vi "AddToCollection.vi"(8 "error in (no error)":errorcluster, 10 "IRenderable":refnum<class "IRenderable.lvclass">, 11 "Collection in":refnum<class "Collection.lvclass">) -> (0 "error out":errorcluster, 3 "Collection out":refnum<class "Collection.lvclass">)   [LabVIEW 2021, in "Markdown.lvlib" / "Collection.lvclass"]
uses:
  Collection.lvclass
  IRenderable/IRenderable.lvclass
  Collection.lvclass/Collection.ctl
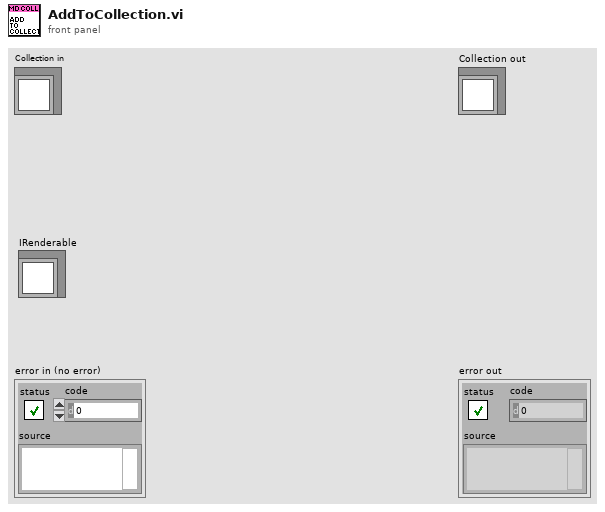
[diagram p1: front panel]
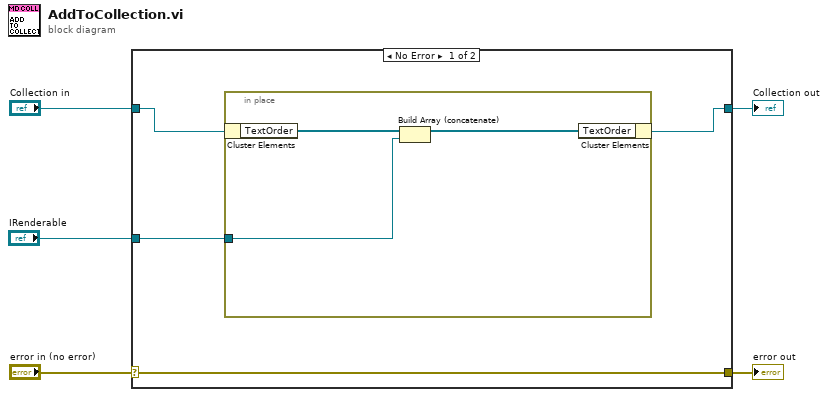
[diagram p0: block diagram]
diagram:
  n1 = case shown="No Error" "error in (no error)" {
    selector: "error in (no error)" -> [w9 w14]
    tunnel: [w9 w14] -> w4
    tunnel: [w6 w13] -> w2
    tunnel: "Collection in" -> [w8 w13]
    tunnel: "IRenderable" -> [w7 _]
    frame No Error {
      n2 = in-place {
        in-place-border: w7 -> [w10]
        n3 = in-place-cluster #1(w8) -> ("TextOrder"=w12:refnum<class "IRenderable.lvclass">[])
        n4 = Build Array (concatenate)(w12, w10) -> (w11:refnum<class "IRenderable.lvclass">[])
        n5 = in-place-cluster #1("TextOrder"=w11) -> (w6:refnum<class "Collection.lvclass">)
      }
    }
    frame Error {
    }
  }
  "error out" <- w4
  "Collection out" <- w2
